vi "Set Session.vi"(8 "error in (no error)":errorcluster, 10 "session handle":T1, 11 "WebDAV in":refnum<class "WebDAV.lvclass">) -> (0 "error out":errorcluster, 3 "WebDAV out":refnum<class "WebDAV.lvclass">)   [LabVIEW 2015, in "RT Management.lvlib" / "WebDAV.lvclass"]
uses:
  WebDAV.lvclass
  <vilib>/WebDAVClient/Advanced/SessionHandle.ctl
  WebDAV.lvclass/WebDAV.ctl
  <vilib>/WebDAVClient/NI_WebDAV.lvlib
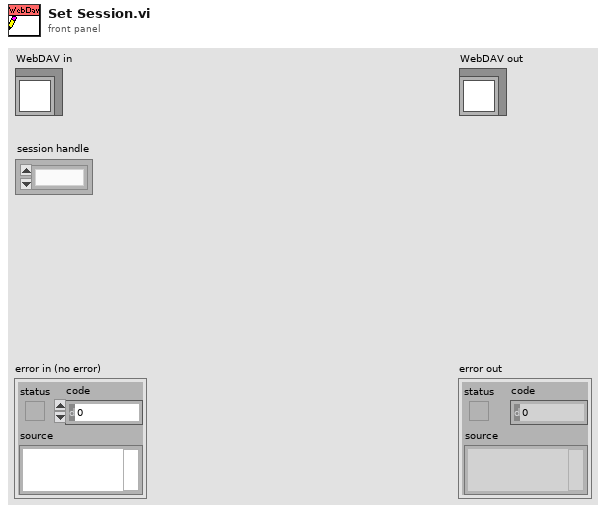
[diagram p1: front panel]
types:
  T1 = typedef "NI_WebDAV.lvlib/SessionHandle.ctl" = refnum<k1>
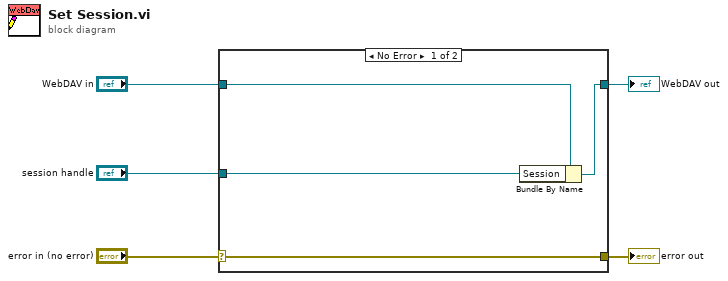
[diagram p0: block diagram]
diagram:
  n1 = case shown="No Error" "error in (no error)" {
    selector: "error in (no error)" -> [w9 w10]
    tunnel: [w9 w10] -> w4
    tunnel: [w7 w11] -> w2
    tunnel: "WebDAV in" -> [w8 w11]
    tunnel: "session handle" -> [w6 _]
    frame No Error {
      n2 = Bundle By Name(cluster=w8, "Session"=w6) -> (w7:refnum<class "WebDAV.lvclass">)
    }
    frame Error {
    }
  }
  "error out" <- w4
  "WebDAV out" <- w2
